vi "221006_Pt100_Kennlinie.vi"(2 "error in (no error)":errorcluster, 3 "B-const.":dbl=-5.7e-07, 4 "A-const.":dbl=0.0039, 5 "Array in":dbl[](array[numeric])=[101.0, 101.0, 118.0, 109.0, 94.0, 114.0, 119.0, 96.0, 113.0, 115.0]) -> (0 "error out":errorcluster={"status"=TRUE, "code"=-9, "source"="221006_Pt100_Kennlinie.vi<ERR>\nNaN calculated in Pt100_Kennlinie.vi\n\n\n<b>Complete call chain:</b>\r\n     221006_Pt100_Kennlinie.vi\r\n     220929_MathNode.vi"}, 1 "Array out":dbl[](array[numeric])=[1.6013546166414365, 1.6013546166414365, 6.793735282183682, 4.80391769163152, nan, 5.9915199725215125, 6.979897481826753, nan, 5.773575769281812, 6.201809806814043])   [LabVIEW 2022 SP3]
doc: "Berechnet die Temperatur aus dem Ohmschen Widerstand Array in. A und B sind konstanten die vom Widerstandsthermometer abhängig sind. Ergebnis NaN führt zu einer Fehlermeldung."
uses:
  <vilib>/Utility/error.llb/Error Cluster From Error Code.vi
  <vilib>/ErrorRing/Error Ring.xnode
panel:
  in  "R0":dbl=100.0
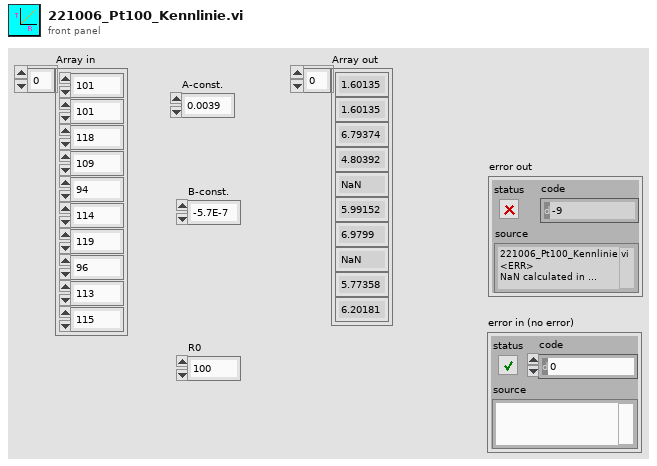
[diagram p1: front panel]
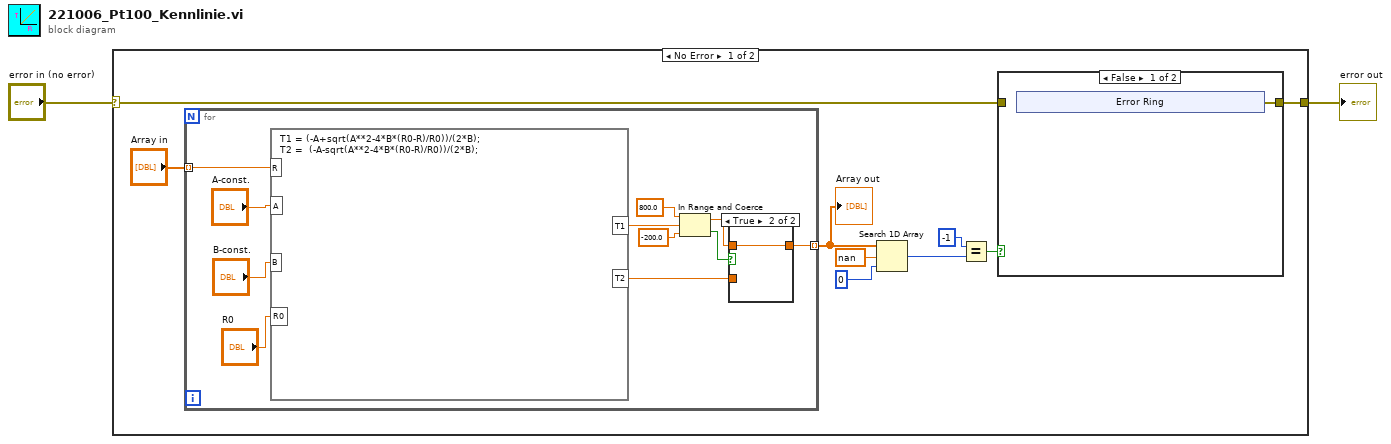
[diagram p0: block diagram]
diagram:
  n1 = case shown="No Error" "error in (no error)" {
    selector: "error in (no error)" -> [w4 w32]
    tunnel: [w3 w32] -> w1
    frame No Error {
      n2 = for {
        tunnel: "Array in" -> [w29] mode=indexing
        tunnel: [w23] -> w10 mode=indexing
        n3 = formula code="T1 = (-A+sqrt(A**2-4*B*(R0-R)/R0))/(2*B);\nT2 =  (-A-sqrt(A**2-4*B*(R0-R)/R0))/(2*B);"("R"=w29, "A"="A-const.", "B"="B-const.", "R0"="R0") -> ("T1"=w22:dbl, "T2"=w21:dbl)
        n4 = In Range and Coerce(upper limit=800.0, x=w22, lower limit=-200.0) -> (coerced(x)=w24:dbl, In Range?=w25:bool)
        n5 = case shown="True" w25 {
          tunnel: w24 -> [_ w31]
          tunnel: [w30 w31] -> w23
          tunnel: w21 -> [w30 _]
          frame False {
          }
          frame True {
          }
        }
      }
      "Array out" <- w10
      n6 = Search 1D Array(1D array=w10, element=nan, start index (0)=0) -> (index of element=w7:i32)
      n7 = Equal?(x=-1, y=w7) -> (x = y?=w5:bool)
      n8 = case shown="False" w5 {
        tunnel: w4 -> [_ w18]
        tunnel: [w12 w18] -> w3
        frame False {
          n9 = xnode "Error Ring"() -> ("error out"=w12:errorcluster)
        }
        frame True {
        }
      }
    }
    frame Error {
    }
  }
  "error out" <- w1
